vi "System.vi"() -> ()   [LabVIEW 2013]
uses:
  <vilib>/imath/engines/lvmath/Functions/Error Handling/error.ctl
  <vilib>/Analysis/2dsp.llb/Real FFT.vi
  <vilib>/imath/engines/lvmath2/RunTimeEngine/NodeEndStatement/NIMS_NodeEndStatement_Output.vi
  <instcachedir>/0/NIMS_NodeEndStatement_Output_53EC0D466D134D7ABD903AC30B43404B.lvgen/NIMS_NodeEndStatement_Output_53EC0D466D134D7ABD903AC30B43404B_004.vi
  <vilib>/imath/engines/lvmath2/RunTimeEngine/ErrorHandling/NIMS_Finalize Error.vi
  <instrlib>/niUSRP/niUSRP Fetch Rx Data (CDB).vi
  <vilib>/imath/engines/lvmath2/RunTimeEngine/BuiltInFunctions/length/NIMS_length(GV).vi
  <instcachedir>/0/NIMS_length(GV)_08A3D13377FD4E4B96F5795FBF3698FA.lvgen/NIMS_length(GV)_08A3D13377FD4E4B96F5795FBF3698FA_001.vi
  <vilib>/imath/engines/lvmath2/RunTimeEngine/RangeToken/NIMS_Range_R2 - Integer.vi
  <instcachedir>/0/NIMS_Range_R2 - Integer_C51C130E5EA5464EA148B28CDAB9615A.lvgen/NIMS_Range_R2 - Integer_C51C130E5EA5464EA148B28CDAB9615A_000.vi
  <instcachedir>/0/NIMS_NodeEndStatement_Output_53EC0D466D134D7ABD903AC30B43404B.lvgen/NIMS_NodeEndStatement_Output_53EC0D466D134D7ABD903AC30B43404B_014.vi
  <instcachedir>/0/NIMS_NodeEndStatement_Output_53EC0D466D134D7ABD903AC30B43404B.lvgen/NIMS_NodeEndStatement_Output_53EC0D466D134D7ABD903AC30B43404B_011.vi
  <vilib>/imath/engines/lvmath2/RunTimeEngine/IndexRead/NIMS V(S).vi
  <instcachedir>/0/NIMS V(S)_0488751826AF41519A22953C041130DC.lvgen/NIMS V(S)_0488751826AF41519A22953C041130DC_005.vi
  <vilib>/imathl/engines/lvmath/Functions/Error Handling/Create Error.vi
  <vilib>/imath/engines/lvmath2/RunTimeEngine/BuiltInFunctions/abs/NIMS_abs(signed).vi
  <instcachedir>/0/NIMS_abs(signed)_C4FCB8E6058B49B797C7C8D53CA5F6EC.lvgen/NIMS_abs(signed)_C4FCB8E6058B49B797C7C8D53CA5F6EC_002.vi
  <vilib>/imath/engines/lvmath2/RunTimeEngine/Managers/WorkSpace/UID Generator.vi
  <vilib>/imath/engines/lvmath2/RunTimeEngine/Managers/SymbolTable/Clear UID.vi
  <instcachedir>/0/NIMS_NodeEndStatement_Output_53EC0D466D134D7ABD903AC30B43404B.lvgen/NIMS_NodeEndStatement_Output_53EC0D466D134D7ABD903AC30B43404B_000.vi
  <vilib>/imath/engines/lvmath2/RunTimeEngine/BuiltInFunctions/close/NIMS_close(Enums).vi
  <vilib>/imath/engines/lvmath2/RunTimeEngine/IndexRead/NIMS V(R2).vi
  <instcachedir>/0/NIMS V(R2)_C76619605A0E4E9F8B2FA9389712AC47.lvgen/NIMS V(R2)_C76619605A0E4E9F8B2FA9389712AC47_001.vi
  <vilib>/imath/engines/lvmath2/RunTimeEngine/BuiltInFunctions/crosscorr/NIMS_crosscorr(GV,GV,Str).vi
  <instcachedir>/0/NIMS_crosscorr(GV,GV,Str)_7F516622EB1B4986A7D0F3F178AC2F2E.lvgen/NIMS_crosscorr(GV,GV,Str)_7F516622EB1B4986A7D0F3F178AC2F2E_000.vi
  <instcachedir>/0/NIMS_abs(signed)_C4FCB8E6058B49B797C7C8D53CA5F6EC.lvgen/NIMS_abs(signed)_C4FCB8E6058B49B797C7C8D53CA5F6EC_006.vi
  <vilib>/imath/engines/lvmath2/RunTimeEngine/BuiltInFunctions/max/1 input/NIMS_max(RV).vi
  <instcachedir>/0/NIMS_max(RV)_237633DB1D604D5BA7001287DF3C7957.lvgen/NIMS_max(RV)_237633DB1D604D5BA7001287DF3C7957_000.vi
  <instcachedir>/0/NIMS_length(GV)_08A3D13377FD4E4B96F5795FBF3698FA.lvgen/NIMS_length(GV)_08A3D13377FD4E4B96F5795FBF3698FA_002.vi
  <vilib>/imath/engines/lvmath2/RunTimeEngine/RunTimeType/NIMS_RunTimeType_From StrictType (excl LVString).vi
  <instcachedir>/0/NIMS_RunTimeType_From StrictType (excl LVString)_4DEE718D6EB74582AA20236969C084FC.lvgen/NIMS_RunTimeType_From StrictType (excl LVString)_4DEE718D6EB74582AA20236969C084FC_000.vi
  <vilib>/imath/engines/lvmath2/RunTimeEngine/LocalVariableDefStatement/MC_LocalVariableDefStatement_Display.vi
  <vilib>/imath/engines/lvmath2/RunTimeEngine/NonStaticBuiltInFunctions/NIMS_NS_close.vi
  <vilib>/imath/engines/lvmath2/RunTimeEngine/NonStaticBuiltInFunctions/Manual/NIMS_NS_figure.vi
  <vilib>/imath/engines/lvmath2/RunTimeEngine/NonStaticBuiltInFunctions/NIMS_NS_crosscorr.vi
  <vilib>/imath/engines/lvmath2/RunTimeEngine/NonStaticBuiltInFunctions/NIMS_NS_abs.vi
  <vilib>/imath/engines/lvmath2/RunTimeEngine/NonStaticBuiltInFunctions/Manual/NIMS_NS_plot.vi
  <vilib>/imath/engines/lvmath2/RunTimeEngine/NonStaticBuiltInFunctions/Manual/NIMS_NS_title.vi
  <vilib>/imath/engines/lvmath2/RunTimeEngine/NonStaticBuiltInFunctions/NIMS_NS_length.vi
  <vilib>/imath/engines/lvmath2/RunTimeEngine/NonStaticBuiltInFunctions/NIMS_NS_real.vi
  <vilib>/imath/engines/lvmath2/RunTimeEngine/NonStaticBuiltInFunctions/NIMS_NS_max.vi
  <vilib>/imath/engines/lvmath2/RunTimeEngine/NonStaticBuiltInFunctions/Manual/NIMS_NS_load.vi
  <vilib>/imath/engines/lvmath2/RunTimeEngine/NonStaticBuiltInFunctions/NIMS_NS_sum.vi
  <vilib>/imath/engines/lvmath2/RunTimeEngine/Managers/SymbolTable/Write Variable.vi
  <vilib>/imath/engines/lvmath2/RunTimeEngine/RunTimeSymbolToken/NIMS_RunTimeSymbolToken_ResolveSymbol.vi
  <instcachedir>/0/NIMS_RunTimeSymbolToken_ResolveSymbol_F94DACEDB8D84373A3303A9E667D843C.lvgen/NIMS_RunTimeSymbolToken_ResolveSymbol_F94DACEDB8D84373A3303A9E667D843C_001.vi
  <instcachedir>/0/NIMS_RunTimeSymbolToken_ResolveSymbol_F94DACEDB8D84373A3303A9E667D843C.lvgen/NIMS_RunTimeSymbolToken_ResolveSymbol_F94DACEDB8D84373A3303A9E667D843C_002.vi
  <vilib>/imath/engines/lvmath2/RunTimeEngine/RunTimeSymbolToken/NIMS_RunTimeSymbolToken_ReadVariable-1out.vi
  <vilib>/imath/engines/lvmath/Functions/Error Handling/MergeErrorsWrapper.vi
  <vilib>/imath/engines/lvmath2/RunTimeEngine/Managers/SymbolTable/Read Variable.vi
  <vilib>/imath/engines/lvmath2/RunTimeEngine/ArithmeticOperatorToken/NIMS_NS_ArithmeticOperator_multmx.vi
  <vilib>/imath/engines/lvmath2/RunTimeEngine/ArithmeticOperatorToken/NIMS_NS_ArithmeticOperator_minus.vi
  <vilib>/imath/engines/lvmath2/RunTimeEngine/ArithmeticOperatorToken/NIMS_NS_ArithmeticOperator_plus.vi
  <vilib>/imath/engines/lvmath2/RunTimeEngine/RowToken/NIMS_RowToken-nonstatic.vi
  <vilib>/imath/engines/lvmath2/RunTimeEngine/MatrixToken/NIMS_MatrixToken-nonstatic.vi
  <vilib>/imath/engines/lvmath2/RunTimeEngine/ArithmeticOperatorToken/NIMS_NS_ArithmeticOperator_rightdivmx.vi
  <vilib>/imath/engines/lvmath2/RunTimeEngine/LastElementToken/NIMS_NS_LastElementToken_Only.vi
  <vilib>/imath/engines/lvmath2/RunTimeEngine/RangeToken/NIMS_NS_Range - 2 inputs.vi
  <vilib>/imath/engines/lvmath2/RunTimeEngine/RunTimeSymbolToken/NIMS_RunTimeSymbolToken_ResolveUDForVariable-1out.vi
  <vilib>/imath/engines/lvmath2/RunTimeEngine/RunTimeType/NIMS_RunTimeType_Get Case Value.vi
  <vilib>/imath/engines/lvmath2/RunTimeEngine/CommandStatement/NIMS_CommandStatement_MaskErr.vi
  <instcachedir>/0/NIMS_RunTimeSymbolToken_ResolveSymbol_F94DACEDB8D84373A3303A9E667D843C.lvgen/NIMS_RunTimeSymbolToken_ResolveSymbol_F94DACEDB8D84373A3303A9E667D843C_003.vi
  <vilib>/imath/engines/lvmath2/RunTimeEngine/NodeEndStatement/MC_NodeEndStatement_Dispose.vi
  <instcachedir>/0/NIMS_NodeEndStatement_Output_53EC0D466D134D7ABD903AC30B43404B.lvgen/NIMS_NodeEndStatement_Output_53EC0D466D134D7ABD903AC30B43404B_003.vi
  <vilib>/imath/engines/lvmath2/RunTimeEngine/RunTimeType/NIMS_RunTimeType_To Numeric.vi
  <instcachedir>/0/NIMS_RunTimeType_To Numeric_4795FB10E831402FABFA341B47E20681.lvgen/NIMS_RunTimeType_To Numeric_4795FB10E831402FABFA341B47E20681_000.vi
  <vilib>/imath/engines/lvmath/Plug In/_Char/RunTimeType/NIMS_CH_RunTimeType_To Character 2D.vi
  <vilib>/imath/engines/lvmath/Plug In/_PlotObject/RunTimeType/NIMS_PO_RunTimeType_To Plot object 2D.vi
  <instcachedir>/0/NIMS_RunTimeType_To Numeric_4795FB10E831402FABFA341B47E20681.lvgen/NIMS_RunTimeType_To Numeric_4795FB10E831402FABFA341B47E20681_001.vi
  <vilib>/imath/engines/lvmath2/RunTimeEngine/CommandStatement/MC_CommandStatement_break.vi
  <vilib>/imath/engines/lvmath2/RunTimeEngine/NonStaticBuiltInFunctions/NIMS_NS_min.vi
  <vilib>/imath/engines/lvmath2/RunTimeEngine/LoopVariableIndexToken/NIMS_NS_LoopVariableIndexToken_Index.vi
  <vilib>/imath/engines/lvmath/Plug In/_Char/NIMS_CH_Character 2D to U8 2D.vi
  <vilib>/Analysis/NI_AALPro.lvlib
  <vilib>/imath/engines/lvmath2/RunTimeEngine/Managers/SymbolTable/NIMS_WorkSpace.lvlib
panel:
  out "error":cdb[][](array[numeric])
  out "index_length":i32
  out "x_start":cdb[](array[numeric])
  out "a":cdb[](array[numeric])
  out "index":i32
  in  "stop 2":bool
  out "Waveform Graph 6":dbl[](graph)
  out "Waveform Graph 5":dbl[][](graph)
  out "Waveform Graph 4":dbl[](graph)
  in  "RX number of samples":i64=100000
  out "RX coerced gain":dbl format="%#_6f"
  out "RX coerced IQ rate":dbl=100000.0 format="%#_6p"
  in  "RX gain":dbl format="%#_6f"
  in  "RX IQ rate":dbl=100000.0 format="%#_6p"
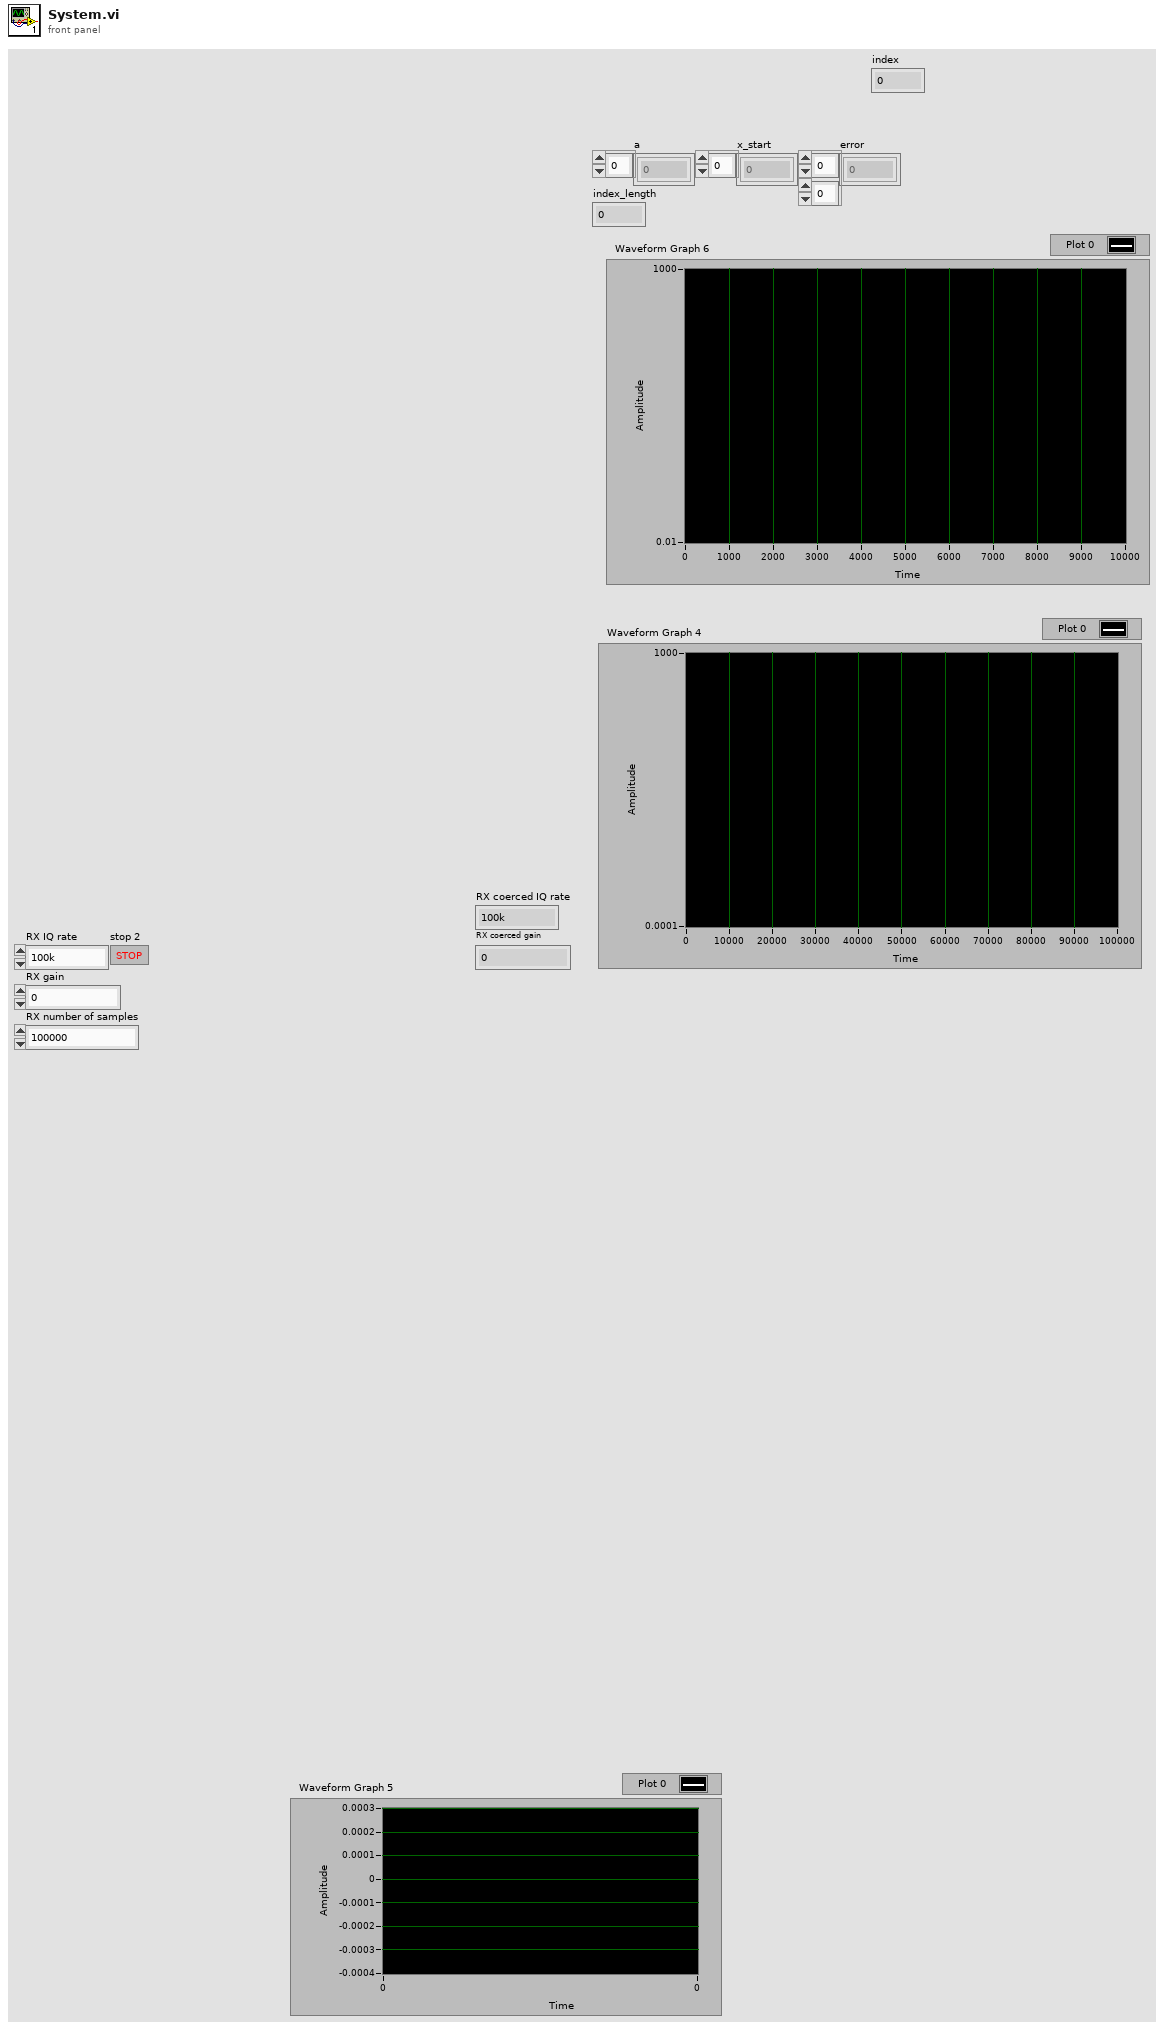
[diagram p1: front panel]
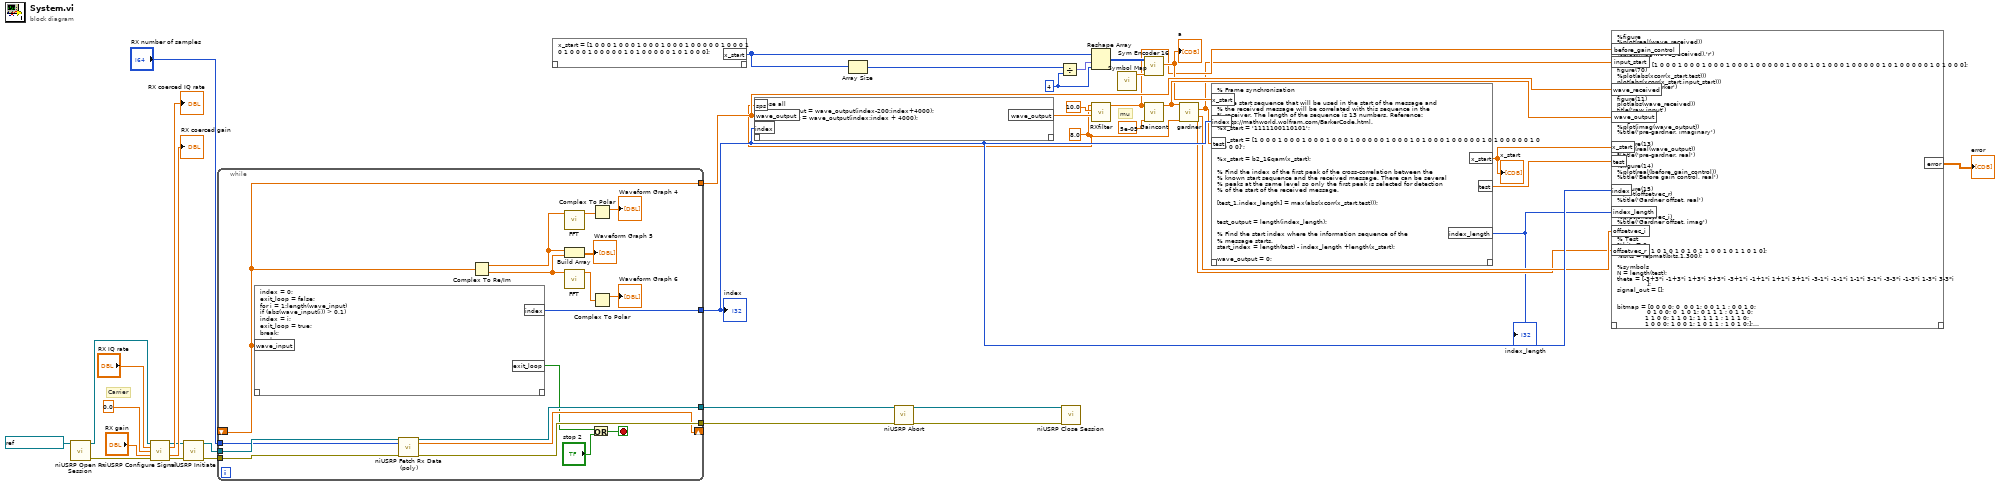
[diagram p0: block diagram]
diagram:
  w14 = 4 ("dimension size")
  w6 = 8.0 ("sps")
  # "mu"
  # "Carrier"
  n1 = call <instrlib>:"niUSRP Open Rx Session.vi"("device names"=refnum<k15> "192.168.10.9") -> ("session handle out"=w38:refnum<k15>, "error out"=w36:errorcluster)  [unwired: 13 in]
  n2 = call <instrlib>:"niUSRP Configure Signal.vi"("session handle"=w38, "IQ rate"="RX IQ rate", "carrier frequency"=0.0, "gain"="RX gain", "error in (no error)"=w36) -> ("session handle out"=w25:refnum<k15>, "coerced IQ rate"=→"RX coerced IQ rate":dbl, "coerced gain"=→"RX coerced gain":dbl, "error out"=w24:errorcluster)  [unwired: 6 in, 1 out]
  n3 = call <instrlib>:"niUSRP Initiate.vi"("session handle"=w25, "error in (no error)"=w24) -> ("session handle out"=w26:refnum<k15>, "error out"=w30:errorcluster)  [unwired: 12 in]
  n4 = while {
    tunnel: w26 -> [w57]
    tunnel: w30 -> [w56]
    tunnel: [w55] -> w29
    tunnel: [w54] -> w28
    tunnel: "RX number of samples" -> [w53]
    shift-right: [w45] -> _
    shift-left: _ -> [w40]
    tunnel: [w44] -> w7
    tunnel: [w40] -> w17
    stop <- w42 stop-if-true
    n5 = mathscript code="index = 0;\nexit_loop = false;\nfor i = 1:length(wave_input)\nif (abs(wave_input(i)) > 0.1)\nindex = i;\nexit_loop = true;\nbreak;\nend\nend"("wave_input"=w40) -> ("index"=w44:i32, "exit_loop"=w41:bool)  [unwired: 1 in, 1 out]
    n6 = call-poly <instrlib>:"niUSRP Fetch Rx Data (poly).vi"("session handle"=w57, "number of samples"=w53, "error in (no error)"=w56) -> ("session handle out"=w55:refnum<k15>, "data"=w45:cdb[], "error out"=w54:errorcluster)  [unwired: 9 in, 1 out]
    n7 = Complex To Re/Im(x + iy=w40) -> (x=w49:dbl[], y=w48:dbl[])
    n8 = call-poly <vilib>:"FFT.vi"("X"=w49) -> ("FFT {X}"=w50:cdb[])  [unwired: 9 in, 1 out]
    n9 = Build Array(w49, w48) -> (→"Waveform Graph 5":dbl[][])
    n10 = call-poly <vilib>:"FFT.vi"("X"=w48) -> ("FFT {X}"=w52:cdb[])  [unwired: 9 in, 1 out]
    n11 = Or(x=w41, y="stop 2") -> (x .or. y?=w42:bool)
    n12 = Complex To Polar(r * e^(i*theta)=w50) -> (r=→"Waveform Graph 4":dbl[])  [unwired: 1 out]
    n13 = Complex To Polar(r * e^(i*theta)=w52) -> (r=→"Waveform Graph 6":dbl[])  [unwired: 1 out]
  }
  "index" <- w7
  n14 = mathscript code="x_start = [1 0 0 0 1 0 0 0 1 0 0 0 1 0 0 0 1 0 0 0 0 0 1 0 0 0 1 0 1 0 0 0 1 0 0 0 0 0 1 0 1 0 0 0 0 0 1 0 1 0 0 0];"() -> ("x_start"=w11:i32[])  [unwired: 1 in, 1 out]
  n15 = mathscript code="close all\n%wave_output = wave_output(index-200:index+4000);\nwave_output = wave_output(index:index + 4000);"("wave_output"=w17, "index"=w7, "sps"=w6) -> ("wave_output"=w20:cdb[])  [unwired: 1 in, 1 out]
  n16 = Array Size(array=w11) -> (size(s)=w12:i32)
  n17 = call <instrlib>:"niUSRP Abort.vi"("session handle"=w29, "error in (no error)"=w28) -> ("session handle out"=w37:refnum<k15>, "error out"=w35:errorcluster)  [unwired: 12 in]
  n18 = Divide(x=w12, y=w14) -> (x/y=w13:fxp<+,27,27>)
  n19 = call <instrlib>:"niUSRP Close Session.vi"("session handle"=w37, "error in (no error)"=w35) -> ()  [unwired: 13 in, 1 out]
  n20 = Reshape Array(w11, w13, w14) -> (w15:i32[][])
  n21 = call "RXfilter.vi"("Array"=w20, "span"=10.0, "sps"=w6) -> ("out"=w8:cdb[])  [unwired: 8 in]
  n22 = call "Symbol Map.vi"() -> ("symbol_map"=w16:cdb[])  [unwired: 11 in]
  n23 = call "Sym Encoder 16.vi"("symbol_map"=w16, "b"=w15) -> ("a"=w10:cdb[])  [unwired: 9 in]
  "a" <- w10
  n24 = call "Gaincont.vi"("mu"=5e-05, "Array"=w8) -> ("out"=w19:cdb[])  [unwired: 9 in]
  n25 = call "gardner.vi"("in"=w19, "sps"=w6) -> ("out"=w4:cdb[], "offsetvec_i"=w3:dbl[], "offsetvec_r"=w2:dbl[])  [unwired: 11 in]
  n26 = mathscript code="% Frame synchronisation\n\n% The start sequence that will be used in the start of the message and\n% the received message will be correlated with this sequence in the \n% receiver. The length of the sequence is 13 numbers. Reference: \n% http://mathworld.wolfram.com/BarkerCode.html.\n%x_start = '1111100110101';\n\n%x_start = [1 0 0 0 1 0 0 0 1 0 0 0 1 0 0 0 1 0 0 0 0 0 1 0 0 0 1 0 1 0 0 0 1 0 0 0 0 0 1 0 1 0 0 0 0 0 1 0 1 0 0 0]';\n\n%x_start = b2_16qam(x_start);\n\n% Find the index of the first peak of the cross-correlation between the \n% known start sequence and the received message. There can be several \n% peaks at the same level so only the first peak is selected for detection \n% of the start of the received message.\n\n[test_1,index_length] = max(abs(xcorr(x_start,test)));\n\n\ntest_output = length(index_length);\n\n% Find the start index where the information sequence of the \n% message starts.\nstart_index = length(test) - index_length +length(x_start);\n\nwave_output = 0;\n\n\ntest = test(start_index:end)"("test"=w4, "index"=w7, "x_start"=w10) -> ("test"=w18:cdb[], "x_start"=w9:cdb[], "index_length"=w1:i32)  [unwired: 1 in, 1 out]
  "x_start" <- w9
  "index_length" <- w1
  n27 = mathscript code="%figure\n%plot(real(wave_received))\n%hold on\n%plot(imag(wave_received),'r')\nclose all\n%x_start = [1 0 0 0 1 0 0 0 1 0 0 0 1 0 0 0 1 0 0 0 0 0 1 0 0 0 1 0 1 0 0 0 1 0 0 0 0 0 1 0 1 0 0 0 0 0 1 0 1 0 0 0];\nfigure(70)\n%plot(abs(xcorr(x_start,test)))\nplot(abs(xcorr(x_start,input_start)))\ntitle('test of barker')\n\nfigure(11)\nplot(abs(wave_received))\ntitle('raw input')\n\n%figure(12)\n%plot(imag(wave_output))\n%title('pre-gardner, imaginary')\n\n%figure(13)\n%plot(real(wave_output))\n%title('pre-gardner, real')\n\n%figure(14)\n%plot(real(before_gain_control))\n%title('Before gain control, real')\n\n%figure(15)\n%plot(offsetvec_r)\n%title('Gardner offset, real')\n\n%figure(16)\n%plot(offsetvec_i)\n%title('Gardner offset. imag')\n\n\n% Test\n%bits = 0;\n%bits = [1 1 0 1 0 1 0 1 0 1 1 0 0 1 0 1 1 0 1 0];\n%bits = repmat(bits,1,300);\n\n%symbols\nN = length(test);\ntheta = [-3+3*i -1+3*i 1+3*i 3+3*i -3+1*i -1+1*i 1+1*i 3+1*i -3-1*i -1-1*i 1-1*i 3-1*i -3-3*i -1-3*i 1-3*i 3-3*i\n               ];\nsignal_out = [];\n\n\nbitmap = [0 0 0 0; 0  0 0 1; 0 0 1 1 ; 0 0 1 0;\n               0 1 0 0; 0  1 0 1; 0 1 1 1 ; 0 1 1 0;\n              1 1 0 0; 1 1 0 1; 1 1 1 1 ; 1 1 1 0;\n              1 0 0 0; 1 0 0 1; 1 0 1 1 ; 1 0 1 0;];\ntheta = theta / max(max(abs(real(theta))));%max(norm(theta));\n\nfigure(313)\n%plot(theta,'*')\n%hold on\nplot(test(100:end),'r*')\n\n\n%bits = bits(index: index + 4000);\n\nfor i = 1:N\n            distance = abs(test(i) - theta);\n   [emp,index_2] =min(distance);\n    \n    signal_out = [signal_out bitmap(index_2,1) bitmap(index_2,2) bitmap(index_2,3) bitmap(index_2,4)];\nend\n\nload 'C:\\Users\\Lab\\Documents\\Projekt\\MATLAB_func\\testvector.mat'\n%test(:,1) = signal_out;\n%test(:,2) = bits;\ntest_2 = bits;\n%test(:,2) = bits;\n\nr1 = bits;\nr2 = signal_out;\nr3 = test;\n\nindex_test = index_length + index;\n\nerror = sum(abs(bits(index_test:index_test) - signal_out));\n\n\n\nfigure(70)\n%plot(abs(xcorr(x_start,test)))\nplot(abs(xcorr(x_start,input_start)))\ntitle('test of barker')\n\nfigure(95)\nplot(test(50:end))\ntitle('test result')\n\nfigure(951)\nplot(test(50:end),'.')"("wave_received"=w17, "wave_output"=w19, "test"=w18, "x_start"=w9, "input_start"=w4, "before_gain_control"=w8, "index"=w7, "offsetvec_i"=w3, "offsetvec_r"=w2, "index_length"=w1) -> ("error"=→"error":cdb[][])  [unwired: 1 in, 1 out]
